vi "NI 9260 Synchronization (Host).vi"(11 "Resource name":T4="RIO0") -> ()   [LabVIEW 2021]
uses:
  <vilib>/rvi/interface/nirviOpenFPGA/nirviOpenFPGA.xnode
  <vilib>/rvi/interface/nirviCloseFPGA/nirviCloseFPGA.xnode
  <vilib>/rvi/interface/nirviReadWriteControl/nirviReadWriteControl.xnode
  <vilib>/rvi/interface/Simulation/niFpgaSimulationCallBeginRW.vi
  <vilib>/rvi/errors/niLvFpgaAdjustHostInterfaceError.vi
  <vilib>/rvi/interface/nirviMethod/nirviMethod.xnode
  <vilib>/FPGAPlugInAG/Dynamic/niLvFpga_WriteFifo_Dynamic.vi
  <vilib>/rvi/errors/niLvFpgaMergeErrorWithErrorCode.vi
  <vilib>/FPGAPlugInAG/Dynamic/niLvFpga_Run_Dynamic.vi
  <vilib>/FPGAPlugInAG/Dynamic/niLvFpga_ConfigureFifo_Dynamic.vi
  NiFpgaLv.dll
  <vilib>/Utility/error.llb/Error Cluster From Error Code.vi
  <vilib>/FPGAPlugInAG/Dynamic/niLvFpga_Close_Dynamic.vi
  <vilib>/FPGAPlugInAG/Dynamic/niLvFpga_ReadFifo_Dynamic.vi
  FPGA Bitfiles/crio-ni9260_FPGATarget_NI9260Synchroniz_8mHRFd2dl5A.lvbitx
  NI 9260 Synchronization (FPGA).vi
  <vilib>/FPGAPlugInAG/cRIO-9053/niLvFpga_Open_cRIO-9053.vi
  <vilib>/rvi/interface/common/dynamic/niFpgaDynamicAddResources.vi
  <vilib>/userDefined/High Color/nirio_resource_hc.ctl
  <vilib>/LabVIEW Targets/FPGA/cRIO/shared/nicrio_ModuleControls/nicrio_cRIO-9260_DataRatesRing2.ctl
  <vilib>/LabVIEW Targets/FPGA/cRIO/shared/nicrio_ModuleControls/nicrio_cRIO-9230_DataRatesRing2.ctl
panel:
  in  "NI 9230 Data Rate":T1=10 items=["12.800 kS/s (NI 9230)"=10, "11.378 kS/s (NI 9230)"=36, "10.240 kS/s (NI 9230)"=21, "9.309 kS/s (NI 9230)"=44, "8.533 kS/s (NI 9230)"=14, "7.877 kS/s (NI 9230)"=52, "7.314 kS/s (NI 9230)"=29, "6.827 kS/s (NI 9230)"=60, "6.400 kS/s (NI 9230)"=18, "6.024 kS/s (NI 9230)"=68, "5.689 kS/s (NI 9230)"=37, "5.389 kS/s (NI 9230)"=76, "5.120 kS/s (NI 9230)"=22, "4.876 kS/s (NI 9230)"=84, "4.655 kS/s (NI 9230)"=45, "4.452 kS/s (NI 9230)"=92, "4.267 kS/s (NI 9230)"=26, "4.096 kS/s (NI 9230)"=100, "3.938 kS/s (NI 9230)"=53, "3.657 kS/s (NI 9230)"=30, "3.413 kS/s (NI 9230)"=61, "3.200 kS/s (NI 9230)"=34, "3.012 kS/s (NI 9230)"=69, "2.844 kS/s (NI 9230)"=38, "2.695 kS/s (NI 9230)"=77, "2.560 kS/s (NI 9230)"=42, "2.438 kS/s (NI 9230)"=85, "2.327 kS/s (NI 9230)"=46, "2.226 kS/s (NI 9230)"=93, "2.133 kS/s (NI 9230)"=50, "2.048 kS/s (NI 9230)"=101, "1.969 kS/s (NI 9230)"=54, "1.829 kS/s (NI 9230)"=58, "1.707 kS/s (NI 9230)"=62, "1.600 kS/s (NI 9230)"=66, "1.506 kS/s (NI 9230)"=70, "1.422 kS/s (NI 9230)"=74, "1.347 kS/s (NI 9230)"=78, "1.280 kS/s (NI 9230)"=82, "1.219 kS/s (NI 9230)"=86, "1.164 kS/s (NI 9230)"=90, "1.113 kS/s (NI 9230)"=94, "1.067 kS/s (NI 9230)"=98, "1.024 kS/s (NI 9230)"=102, "0.985 kS/s (NI 9230)"=106]
  in  "NI 9260 Data Rate":T2=1 items=["51.200 kS/s (NI 9260)"=1, "25.600 kS/s (NI 9260)"=2, "17.067 kS/s (NI 9260)"=3, "12.800 kS/s (NI 9260)"=4, "10.240 kS/s (NI 9260)"=5, "8.533 kS/s (NI 9260)"=6, "7.314 kS/s (NI 9260)"=7, "6.400 kS/s (NI 9260)"=8, "5.689 kS/s (NI 9260)"=9, "5.120 kS/s (NI 9260)"=10, "4.654 kS/s (NI 9260)"=11, "4.267 kS/s (NI 9260)"=12, "3.938 kS/s (NI 9260)"=13, "3.657 kS/s (NI 9260)"=14, "3.413 kS/s (NI 9260)"=15, "3.200 kS/s (NI 9260)"=16, "3.012 kS/s (NI 9260)"=17, "2.845 kS/s (NI 9260)"=18, "2.695 kS/s (NI 9260)"=19, "2.560 kS/s (NI 9260)"=20, "2.438 kS/s (NI 9260)"=21, "2.328 kS/s (NI 9260)"=22, "2.226 kS/s (NI 9260)"=23, "2.133 kS/s (NI 9260)"=24, "2.048 kS/s (NI 9260)"=25, "1.969 kS/s (NI 9260)"=26, "1.896 kS/s (NI 9260)"=27, "1.829 kS/s (NI 9260)"=28, "1.765 kS/s (NI 9260)"=29, "1.707 kS/s (NI 9260)"=30, "1.652 kS/s (NI 9260)"=31]
  out "Analog Input":waveform(dbl)[](graph)
  out "NI 9234 FIFO Time Out":bool
  in  "Host Loop Rate (ms)":u32=100
  out "NI 9260 FIFO Time Out":bool
  in  "Sine Waveform Settings":T3(array[cluster])=[{"Frequency (Hz)"=100.0, "Amplitude (V)"=3.0, "Offset (V)"=0.0, "Phase (deg)"=0.0}, {"Frequency (Hz)"=100.0, "Amplitude (V)"=3.0, "Offset (V)"=0.0, "Phase (deg)"=0.0}]
  in  "stop":bool
  out "FPGA Error out":errorcluster
  in  "Number of Samples per channel":dbl=2048.0 format="%.4p"
  out "Analog Output":waveform(dbl)[](graph)
  out "Host Error out":errorcluster
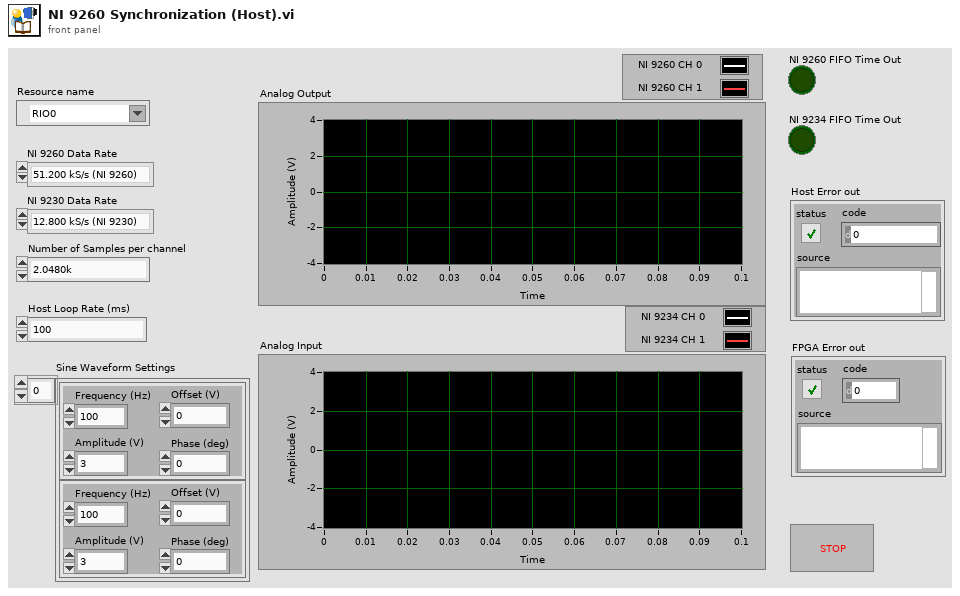
[diagram p1: front panel]
types:
  T1 = typedef "nicrio_cRIO-9230_DataRatesRing2.ctl" = u8
  T2 = typedef "nicrio_cRIO-9260_DataRatesRing2.ctl" = u8
  T3 = cluster{"Frequency (Hz)":dbl, "Amplitude (V)":dbl, "Offset (V)":dbl, "Phase (deg)":dbl}[]
  T4 = typedef "nirio_resource_hc.ctl" = tag
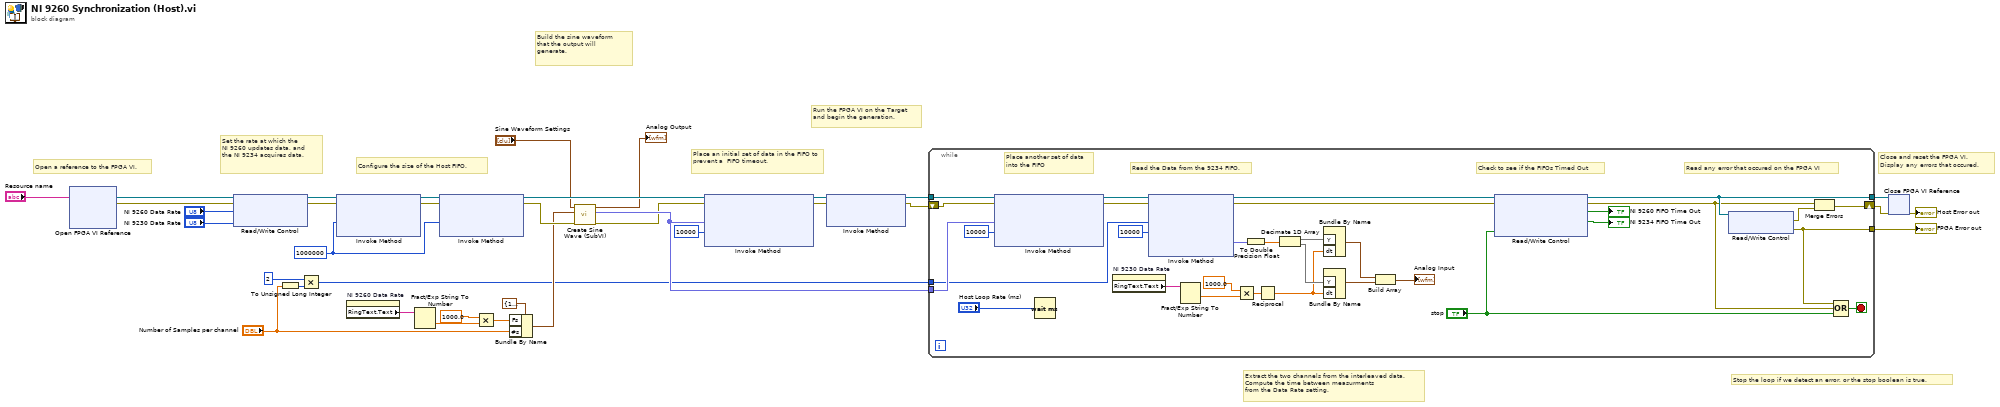
[diagram p0: block diagram]
diagram:
  w4 = u32 1000000 ("Requested Depth")
  # "Build the sine waveform \nthat the output will generate."
  # "Extract the two channels from the interleaved data.\nCompute the time between measurments \nfrom the Data Rate setting."
  # "Place an initial set of data in the FIFO to prevent a  FIFO timeout."
  # "Stop the loop if we detect an error, or the stop boolean is true."
  # "Configure the size of the Host FIFO."
  # "Set the rate at which the \nNI 9260 updates data, and\nthe NI 9234 acquires data."
  # "Close and reset the FPGA VI. \nDisplay any errors that occured."
  # "Run the FPGA VI on the Target and begin the generation."
  # "Open a reference to the FPGA VI."
  n1 = xnode "Open FPGA VI Reference"("resource name"="Resource name") -> ("FPGA VI Reference Out"=w33:refnum<k20>, "error out"=w35:errorcluster)  [unwired: 1 in]
  n2 = xnode "Read/Write Control"("FPGA VI Reference In"=w33, "error in"=w35, "NI 9260 Data Rate"="NI 9260 Data Rate", "NI 9230 Data Rate"="NI 9230 Data Rate") -> ("FPGA VI Reference Out"=w14:refnum<k20>, "error out"=w23:errorcluster)
  n3 = To Unsigned Long Integer(number="Number of Samples per channel") -> (unsigned 32bit integer=w28:u32)
  n4 = Multiply(x=u32 2, y=w28) -> (x*y=w6:u32)
  n5 = xnode "Invoke Method"("FPGA VI Reference In"=w14, "error in"=w23, "Requested Depth"=w4) -> ("FPGA VI Reference Out"=w13:refnum<k20>, "error out"=w15:errorcluster)  [unwired: 1 out]
  n6 = property on="NI 9260 Data Rate" class="Ring (strict)"() -> ("RingText.Text"=w1:string)  [unwired: 2 in, 2 out]
  n7 = Fract/Exp String To Number(string=w1) -> (number=w31:dbl)  [unwired: 3 in, 1 out]
  n8 = xnode "Invoke Method"("FPGA VI Reference In"=w13, "error in"=w15, "Requested Depth"=w4) -> ("FPGA VI Reference Out"=w25:refnum<k20>, "error out"=w12:errorcluster)  [unwired: 1 out]
  n9 = Multiply(x=1000.0, y=w31) -> (x*y=w20:dbl)
  n10 = Bundle By Name(cluster=cluster{"Fs":dbl, "#s":dbl} {"Fs"=1000.0, "#s"=1000.0} ("sampling info"), "Fs"=w20, "#s"="Number of Samples per channel") -> (w10:cluster{"Fs":dbl, "#s":dbl})
  n11 = call "Create Sine Wave (SubVI).vi"("error in (no error)"=w12, "sampling info"=w10, "Sine Waveform Settings"="Sine Waveform Settings") -> ("error out"=w8:errorcluster, "FXP Sinewave"=w9:fxp<+/-,24,4>[], "Voltage Output Waveform"=→"Analog Output":waveform(dbl)[])  [unwired: 6 in]
  n12 = xnode "Invoke Method"("FPGA VI Reference In"=w25, "error in"=w8, "Data"=w9, "Timeout (ms)"=10000) -> ("FPGA VI Reference Out"=w24:refnum<k20>, "error out"=w26:errorcluster)  [unwired: 1 out]
  n13 = xnode "Invoke Method"("FPGA VI Reference In"=w24, "error in"=w26) -> ("FPGA VI Reference Out"=w27:refnum<k20>, "error out"=w7:errorcluster)  [unwired: 1 in]
  n14 = while {
    tunnel: w27 -> [w67]
    tunnel: w9 -> [w66]
    tunnel: [w55] -> w21
    tunnel: [w62] -> w16
    tunnel: w6 -> [w59]
    shift-right: [w41] -> w30
    shift-left: w7 -> [w39]
    stop <- w64 stop-if-true
    # "Check to see if the FIFOs Timed Out"
    # "Read any error that occured on the FPGA VI"
    # "Read the Data from the 9234 FIFO."
    # "Place another set of data\ninto the FIFO"
    n15 = xnode "Invoke Method"("FPGA VI Reference In"=w67, "error in"=w39, "Data"=w66, "Timeout (ms)"=10000) -> ("FPGA VI Reference Out"=w61:refnum<k20>, "error out"=w60:errorcluster)  [unwired: 1 out]
    n16 = Wait (ms)(milliseconds to wait="Host Loop Rate (ms)") -> ()  [unwired: 1 out]
    n17 = property on="NI 9230 Data Rate" class="Ring (strict)"() -> ("RingText.Text"=w36:string)  [unwired: 2 in, 2 out]
    n18 = xnode "Invoke Method"("FPGA VI Reference In"=w61, "error in"=w60, "Number of Elements"=w59, "Timeout (ms)"=10000) -> ("FPGA VI Reference Out"=w57:refnum<k20>, "error out"=w56:errorcluster, "Data"=w54:fxp<+/-,24,7>[])  [unwired: 1 out]
    n19 = Fract/Exp String To Number(string=w36) -> (number=w51:dbl)  [unwired: 4 out]
    n20 = Multiply(x=1000.0, y=w51) -> (x*y=w52:dbl)
    n21 = To Double Precision Float(number=w54) -> (double precision float=w42:dbl[])
    n22 = Reciprocal(x=w52) -> (1/x=w46:dbl)
    n23 = Decimate 1D Array(w42) -> (w48:dbl[], w47:dbl[])
    n24 = Bundle By Name("Y"=w48, "dt"=w46) -> (w50:waveform(dbl))  [unwired: 1 out]
    n25 = Bundle By Name("Y"=w47, "dt"=w46) -> (w49:waveform(dbl))  [unwired: 1 out]
    n26 = Build Array(w50, w49) -> (→"Analog Input":waveform(dbl)[])
    n27 = xnode "Read/Write Control"("FPGA VI Reference In"=w57, "error in"=w56, "stop"="stop") -> ("FPGA VI Reference Out"=w55:refnum<k20>, "error out"=w40:errorcluster, "NI 9260 FIFO Time Out"=→"NI 9260 FIFO Time Out":bool, "NI 9230 FIFO Time Out"=→"NI 9234 FIFO Time Out":bool)
    n28 = xnode "Read/Write Control"("FPGA VI Reference In"=w55) -> ("error out"=w38:errorcluster, "FPGA Error out"=w62:errorcluster)  [unwired: 1 in, 1 out]
    n29 = Merge Errors(w40, w38) -> (w41:errorcluster)
    n30 = Compound Arithmetic op=OR(w62, w40, "stop") -> (w64:bool)
  }
  "FPGA Error out" <- w16
  n31 = xnode "Close FPGA VI Reference"("FPGA VI Reference In"=w21, "error in"=w30) -> ("error out"=→"Host Error out":errorcluster)
